vi "Prog_Revision_Date.vi"(5 "Input string":string) -> (0 "Revision time (s)":u32, 3 "Prog's last revision date":string)   [LabVIEW 2010]
uses:
  <vilib>/Utility/miscctls.llb/LVDateTimeRec.ctl
panel:
  out "time string":string
  out "Input Date string":string
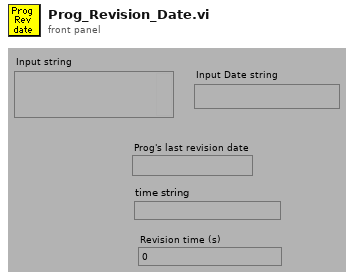
[diagram p1: front panel]
types:
  T1 = typedef "LVDateTimeRec.ctl" = cluster{"fractional second":dbl, "second":i32, "minute":i32, "hour":i32, "day of month":i32, "month":i32, "year":i32, "day of week":i32, "day of year":i32, "DST":i32}
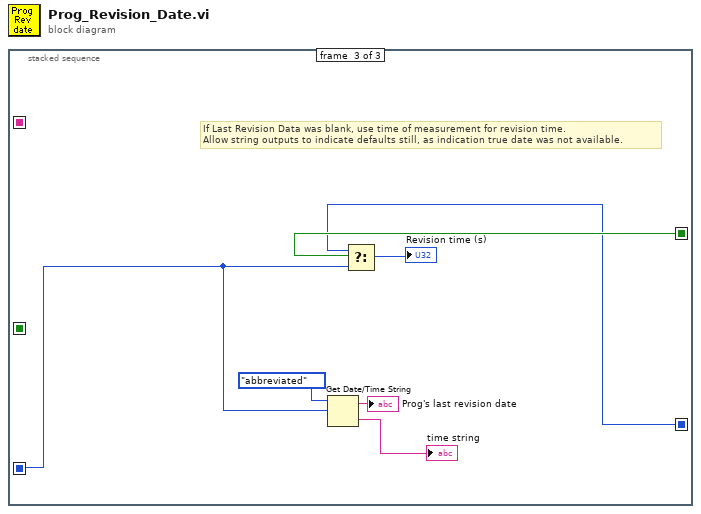
[diagram p0: block diagram]
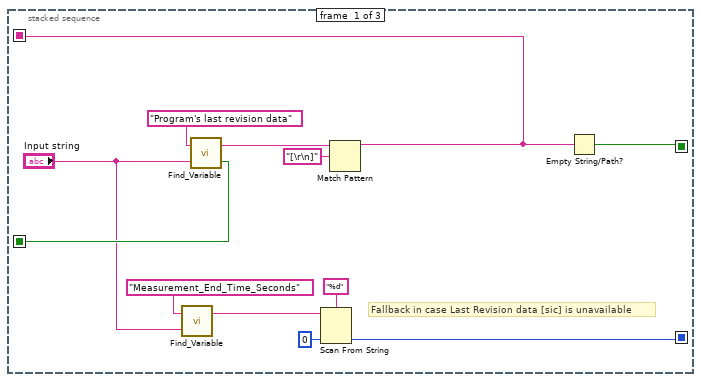
[diagram p2: hidden frame]
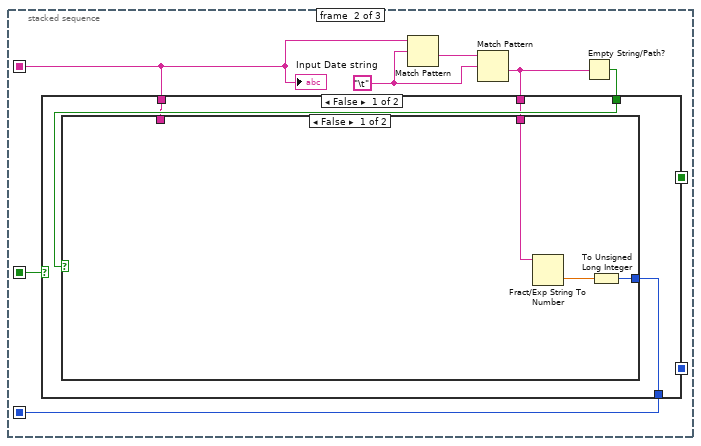
[diagram p3: hidden frame]
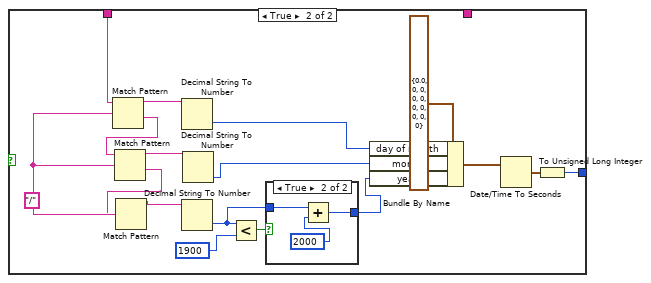
[diagram p4: hidden frame]
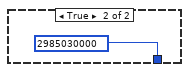
[diagram p6: hidden frame]
diagram:
  n1 = stacked-sequence {
    seq-local: [_ w19 _] -> [_ _ w53]
    seq-local: [w6 _ _] -> [_ w13 _]
    seq-local: [w9 _ _] -> [_ w14 _]
    seq-local: [w5 _ _] -> [_ _ w50]
    seq-local: [w1 _ _] -> [_ _ w49]
    frame #0 {
      # "Fallback in case Last Revision data [sic] is unavailable"
      n2 = call "Find_Variable.vi"("Input string"="Input string", "Variable name"="Measurement_End_Time_Seconds") -> ("After  Matched string"=w3:string)  [unwired: 1 out]
      n3 = call "Find_Variable.vi"("Input string"="Input string", "Variable name"="Program's last revision data") -> ("No Match?"=w9:bool, "After  Matched string"=w11:string)
      n4 = Scan From String(format string="%d", input string=w3, default 1=u32 0 ("default value 1")) -> (output 1=w1:u32)  [unwired: 2 in, 3 out]
      n5 = Match Pattern(string=w11, regular expression="[\r\n]") -> (before substring=w6:string)  [unwired: 4 out]
      n6 = Empty String/Path?(string/path=w6) -> (empty?=w5:bool)
    }
    frame #1 {
      w18 = "\t"
      n7 = Match Pattern(string=w13, regular expression=w18) -> (after substring=w17:string)  [unwired: 4 out]
      n8 = Match Pattern(string=w17, regular expression=w18) -> (after substring=w15:string)  [unwired: 4 out]
      n9 = Empty String/Path?(string/path=w15) -> (empty?=w16:bool)
      n10 = case shown="False" w14 {
        tunnel: [w23 u32 2985030000 ("seconds")] -> w19
        tunnel: w16 -> [w22 _]
        tunnel: w15 -> [w21 _]
        tunnel: w13 -> [w20 _]
        frame False {
          n11 = case shown="False" w22 {
            tunnel: [w24 w35] -> w23
            tunnel: w21 -> [w26 _]
            tunnel: w20 -> [_ w29]
            frame False {
              n12 = Fract/Exp String To Number(string=w26) -> (number=w25:dbl)  [unwired: 4 out]
              n13 = To Unsigned Long Integer(number=w25) -> (unsigned 32bit integer=w24:u32)
            }
            frame True {
              w41 = "/" ("search char (-)")
              n14 = Match Pattern(string=w29, regular expression=w41) -> (before substring=w40:string, after substring=w39:string)  [unwired: 3 out]
              n15 = Match Pattern(string=w39, regular expression=w41) -> (before substring=w38:string, after substring=w36:string)  [unwired: 3 out]
              n16 = Match Pattern(string=w36, regular expression=w41) -> (before substring=w37:string)  [unwired: 4 out]
              n17 = Decimal String To Number(string=w40) -> (number=w43:i32)  [unwired: 3 out]
              n18 = Decimal String To Number(string=w37) -> (number=w31:i32)  [unwired: 3 out]
              n19 = Decimal String To Number(string=w38) -> (number=w42:i32)  [unwired: 3 out]
              n20 = Less?(x=w31, y=1900) -> (x < y?=w32:bool)
              n21 = case shown="True" w32 {
                tunnel: w31 -> [w44 w46]
                tunnel: [w44 w45] -> w30
                frame False {
                }
                frame True {
                  n22 = Add(x=w46, y=2000) -> (x+y=w45:i32)
                }
              }
              n23 = Bundle By Name(cluster=T1 {"fractional second"=0.0, "second"=0, "minute"=0, "hour"=0, "day of month"=0, "month"=0, "year"=0, "day of week"=0, "day of year"=0, "DST"=0} ("date time rec"), "day of month"=w43, "month"=w42, "year"=w30) -> (w27:T1)
              n24 = Date/Time To Seconds(2:w27) -> (0:w34:timestamp)  [unwired: 1 in]
              n25 = To Unsigned Long Integer(number=w34) -> (unsigned 32bit integer=w35:u32)
            }
          }
        }
        frame True {
        }
      }
      "Input Date string" <- w13
    }
    frame #2 {
      # "If Last Revision Data was blank, use time of measurement for revision time.\nAllow string outputs to indicate defaults still, as indication true date was not available."
      n26 = Get Date/Time String(date format (0)=enum16{"short", "long", "abbreviated"}."abbreviated", seconds (now)=w53) -> (date string=→"Prog's last revision date":string, time string=→"time string":string)  [unwired: 1 out]
      n27 = Select(t=w49, s=w50, f=w53) -> (s? t:f=→"Revision time (s)":u32)
    }
  }
